vi "datasetDescription.set.vi"(8 "error in (no error)":errorcluster, 10 "datasetDescription":string, 11 "dataset in":refnum<class "dataset.lvclass">) -> (0 "error out":errorcluster, 3 "dataset out":refnum<class "dataset.lvclass">)   [LabVIEW 2020, in "datasources.lvlib" / "dataset.lvclass"]
uses:
  dataset.lvclass
  dataset.lvclass/dataset.ctl
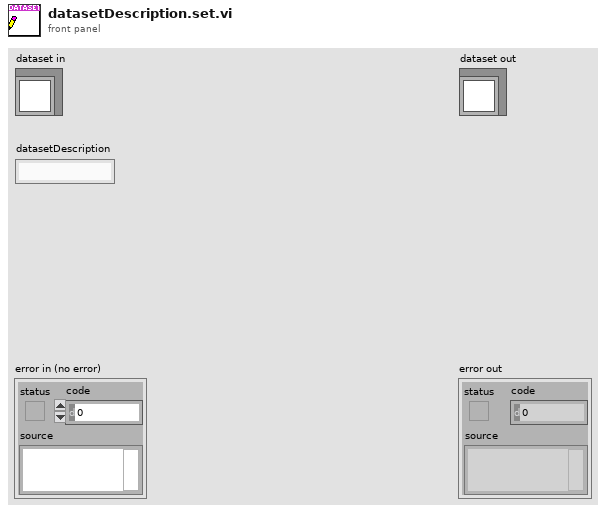
[diagram p1: front panel]
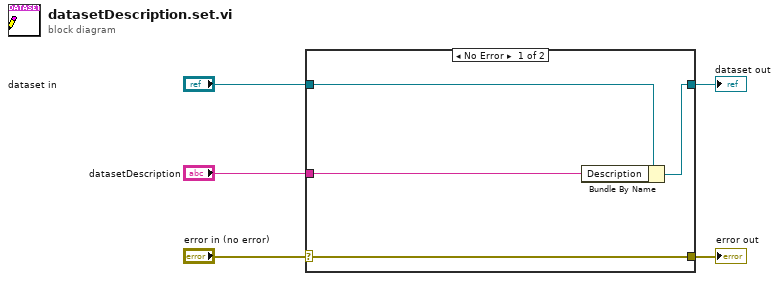
[diagram p0: block diagram]
diagram:
  n1 = case shown="No Error" "error in (no error)" {
    selector: "error in (no error)" -> [w9 w10]
    tunnel: [w9 w10] -> w4
    tunnel: [w7 w11] -> w2
    tunnel: "dataset in" -> [w8 w11]
    tunnel: "datasetDescription" -> [w6 _]
    frame No Error {
      n2 = Bundle By Name(cluster=w8, "Description"=w6) -> (w7:refnum<class "dataset.lvclass">)
    }
    frame Error {
    }
  }
  "error out" <- w4
  "dataset out" <- w2
